vi "Westcoast Drive Begin.vi"   [LabVIEW 2018]
uses:
  <vilib>/Rock Robotics/WPI/ThirdParty/REV Robotics/SPARK MAX/Typedef/Spark MAX Motor Type.ctl
  <vilib>/Rock Robotics/WPI/Joystick/WPI_JoystickDeviceEnum.ctl
  <vilib>/Rock Robotics/WPI/Solenoid/WPI_SolenoidChannel.ctl
  <vilib>/Rock Robotics/WPI/Utilities/WPI_GetSetVariantRefNum.vi
  <vilib>/Rock Robotics/WPI/Solenoid/WPI_SolenoidOpenDouble.vi
types:
  T1 = typedef "WPI_SolenoidChannel.ctl" = enum8{"Solenoid 0", "Solenoid 1", "Solenoid 2", "Solenoid 3", "Solenoid 4", "Solenoid 5", "Solenoid 6", "Solenoid 7", "Invalid"}
  T2 = typedef "WPI_JoystickDeviceEnum.ctl" = enum16{"USB 0", "USB 1", "USB 2", "USB 3", "USB 4", "USB 5"}
  T3 = typedef "Spark MAX Motor Type.ctl" = enum16{"Brushed", "Brushless"}
  T4 = typedef "WPI_MotorControlDeviceRef.ctl" = cluster{"DeviceStatus":errorcluster, "Type":T5, "PWM":cluster{"PWM Channel":T6, "DeadBand":T7}, "CAN":cluster{"Device Number":u8, "SetOutput VI Ref":variant, "GetOutput VI Ref":variant, "Enable VI Ref":variant, "Disable VI Ref":variant, "Data":variant}, "Invert":bool, "DIO PWM":cluster{"PWM \"Enable\" Channel":T6, "DIOChannel":T8, "PWM Rate":dbl}}
  T5 = typedef "WPI_MotorControlType.ctl" = enum16{"PWM", "CAN", "DIO PWM"}
  T6 = typedef "FPGA_DIOPWMChannel.ctl" = enum8{"PWM 0", "PWM 1", "PWM 2", "PWM 3", "PWM 4", "PWM 5", "PWM 6", "PWM 7", "PWM 8", "PWM 9", "PWM MXP 0", "PWM MXP 1", "PWM MXP 2", "PWM MXP 3", "PWM MXP 4", "PWM MXP 5", "PWM MXP 6", "PWM MXP 7", "PWM MXP 8", "PWM MXP 9", "Invalid"}
  T7 = typedef "WPI_PWMDeadband.ctl" = cluster{"Name":string, "maxPositivePwm":i32, "minPositivePwm":i32, "centerPwm":i32, "maxNegativePwm":i32, "minNegativePwm":i32, "angularRange":u16}
  T8 = typedef "FPGA_DIOChannel.ctl" = enum8{"DIO 0", "DIO 1", "DIO 2", "DIO 3", "DIO 4", "DIO 5", "DIO 6", "DIO 7", "DIO 8", "DIO 9", "DIO MXP 0", "DIO MXP 1", "DIO MXP 2", "DIO MXP 3", "DIO MXP 4", "DIO MXP 5", "DIO MXP 6", "DIO MXP 7", "DIO MXP 8", "DIO MXP 9", "DIO MXP 10", "DIO MXP 11", "DIO MXP 12", "DIO MXP 13", "DIO MXP 14", "DIO MXP 15", "SPI Port CS1", "SPI Port CS2", "SPI Port CS3", "SPI Port MISO", "SPI Port MOSI", "Invalid"}
  T9 = typedef "WPI_CompressorDevRef.ctl" = cluster{"DevStatus":errorcluster, "Pneumatics Control Module":u8}
  T10 = typedef "WPI_JoystickDevRef.ctl" = cluster{"Device":T2}
  T11 = typedef "WPI_SolenoidDevRef.ctl" = cluster{"DevStatus":errorcluster, "Pneumatics Control Module":u8, "Forward Solenoid Channel":T1, "Reverse Solenoid Channel":T1}
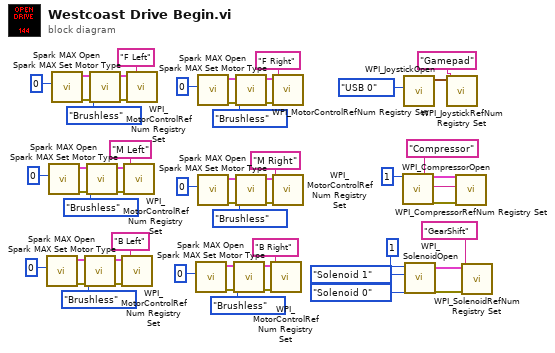
[diagram p0: block diagram]
diagram:
  n1 = call <vilib>:"Spark MAX Open.vi"("Device Number"=u8 0) -> ("error out"=w24:errorcluster, "MotorControlDeviceRef"=w25:T4)  [unwired: 9 in]
  n2 = call <vilib>:"Spark MAX Open.vi"("Device Number"=u8 0) -> ("error out"=w31:errorcluster, "MotorControlDeviceRef"=w32:T4)  [unwired: 9 in]
  n3 = call <vilib>:"Spark MAX Open.vi"("Device Number"=u8 0) -> ("error out"=w52:errorcluster, "MotorControlDeviceRef"=w53:T4)  [unwired: 9 in]
  n4 = call <vilib>:"Spark MAX Set Motor Type.vi"("error in (no error)"=w24, "Enum"=Spark_MAX_Motor_Type."Brushless", "MotorControlDevRef"=w25) -> ("error out"=w21:errorcluster, "MotorControlDeviceRef"=w22:T4)  [unwired: 7 in]
  n5 = call <vilib>:"Spark MAX Set Motor Type.vi"("error in (no error)"=w31, "Enum"=Spark_MAX_Motor_Type."Brushless", "MotorControlDevRef"=w32) -> ("error out"=w28:errorcluster, "MotorControlDeviceRef"=w29:T4)  [unwired: 7 in]
  n6 = call <vilib>:"Spark MAX Set Motor Type.vi"("error in (no error)"=w52, "Enum"=Spark_MAX_Motor_Type."Brushless", "MotorControlDevRef"=w53) -> ("error out"=w49:errorcluster, "MotorControlDeviceRef"=w50:T4)  [unwired: 7 in]
  n7 = call <vilib>:"WPI_MotorControlRefNum Registry Set.vi"("error in (no error)"=w21, "refnum name"="B Left", "MotorControlDevRef"=w22) -> ()  [unwired: 7 in, 2 out]
  n8 = call <vilib>:"WPI_MotorControlRefNum Registry Set.vi"("error in (no error)"=w28, "refnum name"="M Left", "MotorControlDevRef"=w29) -> ()  [unwired: 7 in, 2 out]
  n9 = call <vilib>:"WPI_MotorControlRefNum Registry Set.vi"("error in (no error)"=w49, "refnum name"="F Left", "MotorControlDevRef"=w50) -> ()  [unwired: 7 in, 2 out]
  n10 = call <vilib>:"Spark MAX Open.vi"("Device Number"=u8 0) -> ("error out"=w17:errorcluster, "MotorControlDeviceRef"=w18:T4)  [unwired: 9 in]
  n11 = call <vilib>:"Spark MAX Open.vi"("Device Number"=u8 0) -> ("error out"=w45:errorcluster, "MotorControlDeviceRef"=w46:T4)  [unwired: 9 in]
  n12 = call <vilib>:"Spark MAX Open.vi"("Device Number"=u8 0) -> ("error out"=w38:errorcluster, "MotorControlDeviceRef"=w39:T4)  [unwired: 9 in]
  n13 = call <vilib>:"Spark MAX Set Motor Type.vi"("error in (no error)"=w17, "Enum"=Spark_MAX_Motor_Type."Brushless", "MotorControlDevRef"=w18) -> ("error out"=w14:errorcluster, "MotorControlDeviceRef"=w15:T4)  [unwired: 7 in]
  n14 = call <vilib>:"Spark MAX Set Motor Type.vi"("error in (no error)"=w45, "Enum"=Spark_MAX_Motor_Type."Brushless", "MotorControlDevRef"=w46) -> ("error out"=w42:errorcluster, "MotorControlDeviceRef"=w43:T4)  [unwired: 7 in]
  n15 = call <vilib>:"Spark MAX Set Motor Type.vi"("error in (no error)"=w38, "Enum"=Spark_MAX_Motor_Type."Brushless", "MotorControlDevRef"=w39) -> ("error out"=w35:errorcluster, "MotorControlDeviceRef"=w36:T4)  [unwired: 7 in]
  n16 = call <vilib>:"WPI_MotorControlRefNum Registry Set.vi"("error in (no error)"=w14, "refnum name"="B Right", "MotorControlDevRef"=w15) -> ()  [unwired: 7 in, 2 out]
  n17 = call <vilib>:"WPI_MotorControlRefNum Registry Set.vi"("error in (no error)"=w42, "refnum name"="F Right", "MotorControlDevRef"=w43) -> ()  [unwired: 7 in, 2 out]
  n18 = call <vilib>:"WPI_MotorControlRefNum Registry Set.vi"("error in (no error)"=w35, "refnum name"="M Right", "MotorControlDevRef"=w36) -> ()  [unwired: 7 in, 2 out]
  n19 = call <vilib>:"WPI_CompressorOpen.vi"("Pneumatics Control Module (0)"=u8 1) -> ("CompressorDevRef"=w9:T9, "error out"=w10:errorcluster)  [unwired: 13 in]
  n20 = call <vilib>:"WPI_JoystickOpen.vi"("JoystickDevice"=WPI_JoystickDeviceEnum."USB 0") -> ("JoystickDevRef"=w13:T10)  [unwired: 10 in]
  n21 = call-poly <vilib>:"WPI_SolenoidOpen.vi"("Reverse Solenoid Channel"=WPI_SolenoidChannel."Solenoid 0", "Forward Solenoid Channel"=WPI_SolenoidChannel."Solenoid 1", "Pneumatics Control Module (0)"=u8 1) -> ("error out"=w2:errorcluster, "SolenoidDevRef"=w3:T11)  [unwired: 7 in]
  n22 = call <vilib>:"WPI_JoystickRefNum Registry Set.vi"("refnum name"="Gamepad", "JoystickDevRef"=w13) -> ()  [unwired: 8 in, 2 out]
  n23 = call <vilib>:"WPI_CompressorRefNum Registry Set.vi"("error in (no error)"=w10, "refnum name"="Compressor", "CompressorDevRef"=w9) -> ()  [unwired: 7 in, 2 out]
  n24 = call <vilib>:"WPI_SolenoidRefNum Registry Set.vi"("error in (no error)"=w2, "refnum name"="GearShift", "SolenoidDevRef"=w3) -> ()  [unwired: 7 in, 2 out]
